vi "SetResultManagerInstance.vi"(11 "ResultManager":T1) -> ()   [LabVIEW 2011]
uses:
  qtrk/QTrkLVBinding/ResultManagerInstance.ctl
  SemaphoreResultManager.vi
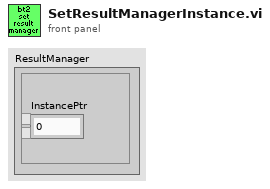
[diagram p1: front panel]
types:
  T1 = typedef "ResultManagerInstance.ctl" = cluster{"InstancePtr":u64}
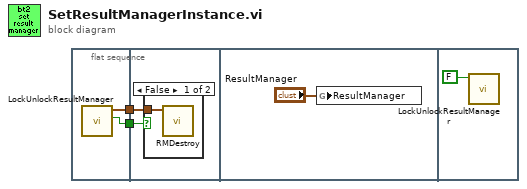
[diagram p0: block diagram]
diagram:
  n1 = flat-sequence {
    tunnel: [w4] -> w2
    tunnel: [w3] -> w1
    tunnel: w2 -> [w6]
    tunnel: w1 -> [w5]
    frame #0 {
      n2 = call "LockUnlockResultManager.vi"() -> ("Valid non-zero instance"=w3:bool, "ResultManager"=w4:T1)  [unwired: 9 in, 1 out]
    }
    frame #1 {
      n3 = case shown="False" w5 {
        tunnel: w6 -> [w7 _]
        frame False {
          n4 = call "RMDestroy.vi"("ResultManager"=w7) -> ()  [unwired: 9 in, 2 out]
        }
        frame True {
        }
      }
    }
    frame #2 {
      n5 = global write "SemaphoreResultManager.vi" "ResultManager"("ResultManager") -> ()
    }
    frame #3 {
      n6 = call "LockUnlockResultManager.vi"("Lock? (T)"=FALSE) -> ()  [unwired: 8 in, 3 out]
    }
  }
